vi "Insert_empty_element_with_zero.vi"(10 "searched date":string[](array[string]), 11 "fixed date":string[](array[string])) -> (3 "O/P":string[](array[string]))   [LabVIEW 2017]
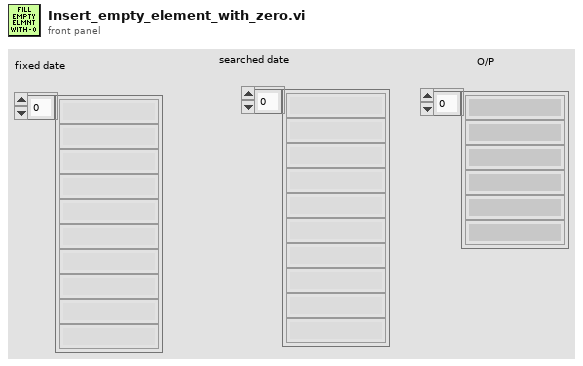
[diagram p1: front panel]
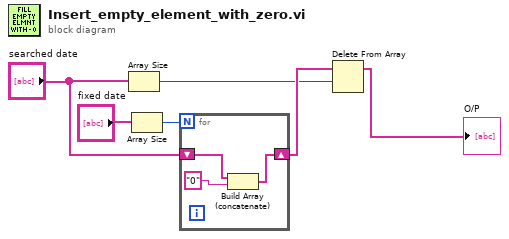
[diagram p0: block diagram]
diagram:
  n1 = Array Size(array="searched date") -> (size(s)=w3:i32)
  n2 = Array Size(array="fixed date") -> (size(s)=w4:i32)
  n3 = for {
    N: w4 -> [_]
    shift-right: [w8] -> w5
    shift-left: "searched date" -> [w9]
    n4 = Build Array (concatenate)(w9, "0") -> (w8:string[])
  }
  n5 = Delete From Array(array=w5, length=w3) -> (array with subset deleted=→"O/P":string[])  [unwired: 1 in, 1 out]
